vi "Calculate_Distance.vi"(0 "Speed":dbl, 1 "Current Distance":dbl, 3 "error in (no error)":errorcluster) -> (8 "New Distance":dbl, 10 "error out":errorcluster)   [LabVIEW 2026]
doc: "Calculate_Distance.vi calculates the new distance travelled every second by adding the user's current speed per second to the current distance."
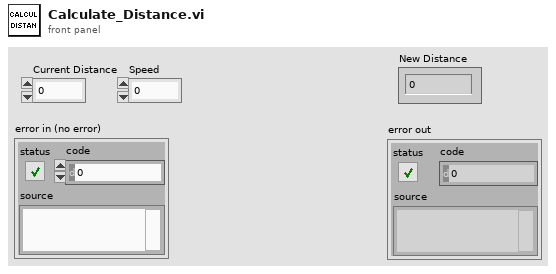
[diagram p1: front panel]
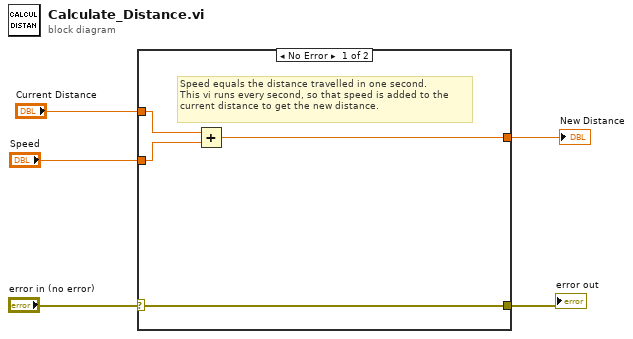
[diagram p0: block diagram]
diagram:
  n1 = case shown="No Error" "error in (no error)" {
    selector: "error in (no error)" -> [w9 w11]
    tunnel: [w9 w11] -> w4
    tunnel: "Current Distance" -> [w8 w10]
    tunnel: "Speed" -> [w7 _]
    tunnel: [w6 w10] -> w1
    frame No Error {
      # "Speed equals the distance travelled in one second.\nThis vi runs every second, so that speed is added to the \ncurrent distance to get the new distance."
      n2 = Add(x=w8, y=w7) -> (x+y=w6:dbl)
    }
    frame Error {
    }
  }
  "New Distance" <- w1
  "error out" <- w4
